vi "ex_Global.vi"() -> ()   [LabVIEW 2018]
panel:
  in  "빈 버튼":bool
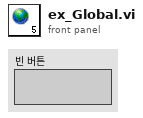
[diagram p1: front panel]
diagram:
